vi "find next node.vi"(8 "error in (no error)":errorcluster, 10 "map":T1[][](array[typedef]), 11 "current_path in":T1[](array[typedef])) -> (0 "error out":errorcluster, 1 "T = a next node was found":bool, 2 "next node":T1, 3 "current_path out":T1[](array[typedef]))   [LabVIEW 2021, in "Project Euler.lvlib"]
uses:
  Project Euler.lvlib
  lattice_path_node.ctl
  lattice_path_direction.ctl
panel:
  out "map no. of columns":i32
  out "map no. of rows":i32
  out "last (most recent) node of path":T1
  # "Development\ncontrols/indicators useful for development and testing, but which are not outputs of the VI"
  # "Input\nInputs to the VI"
  # "Output\nOutputs of the VI"
  # "Description\n\nBlank VI with error handling case. \n\nSummarize the use of this VI in this space."
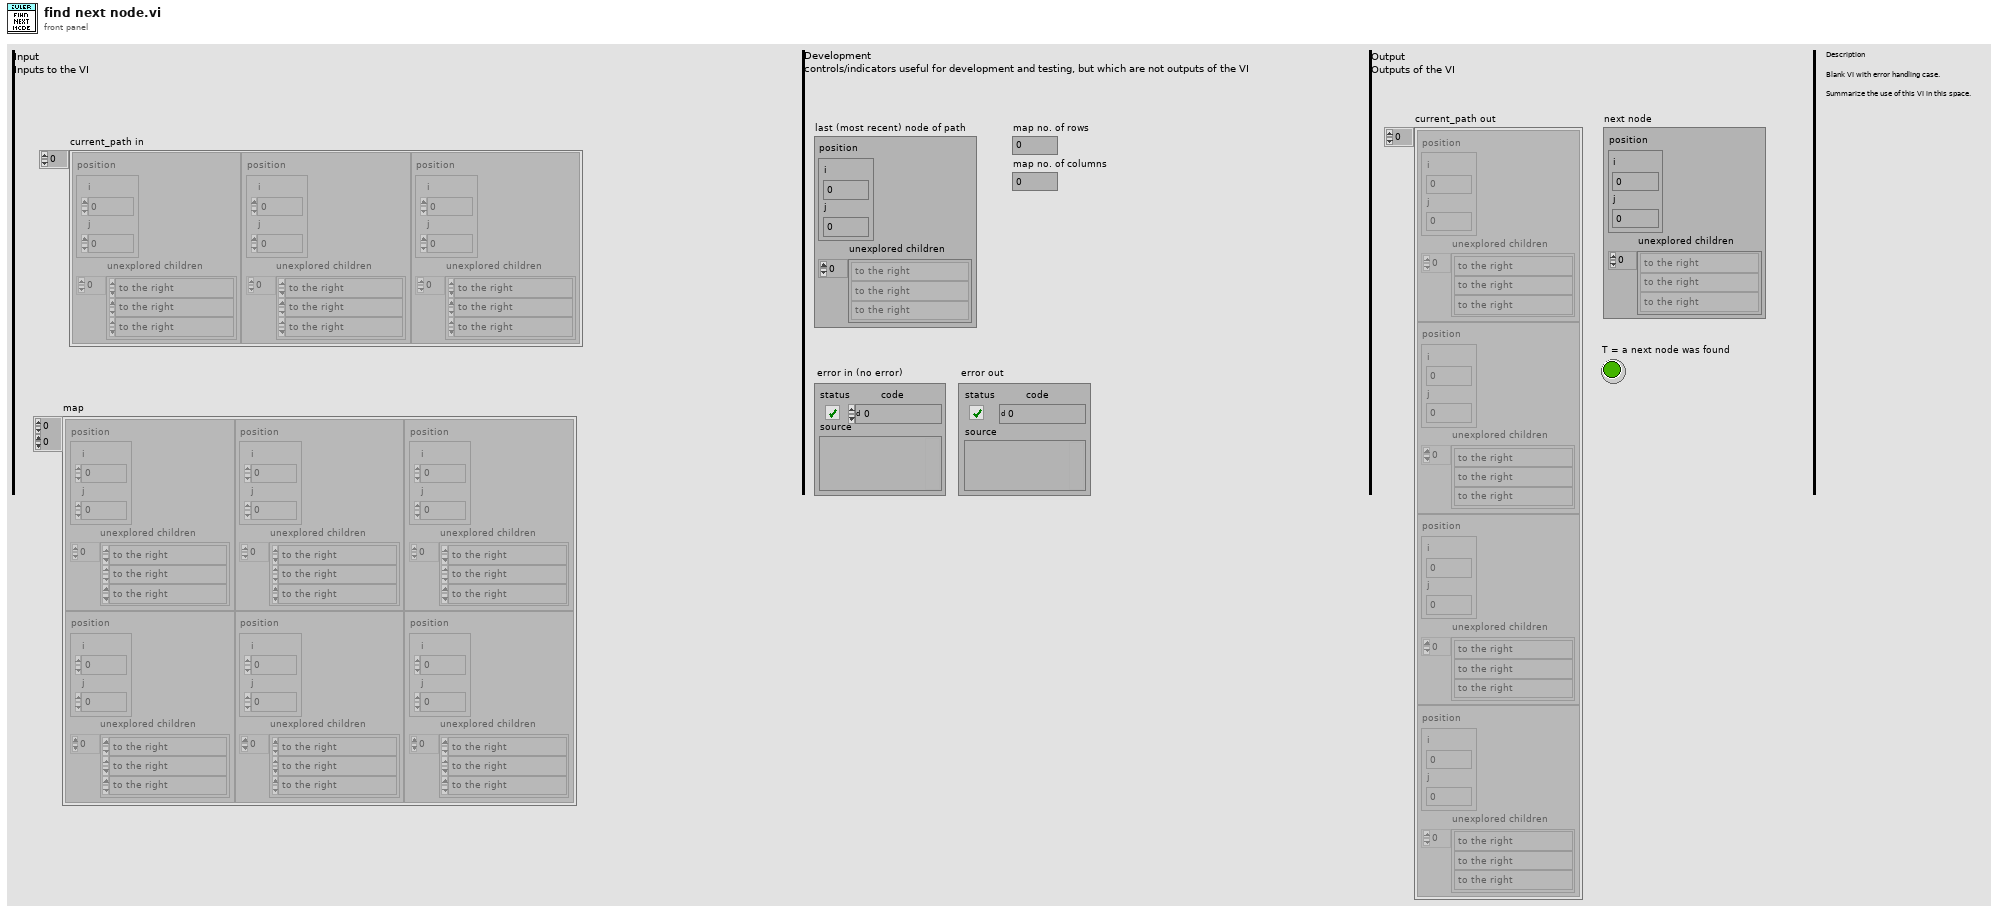
[diagram p1: front panel]
types:
  T1 = typedef "Project Euler.lvlib/lattice_path_node.ctl" = cluster{"position":cluster{"i":i32, "j":i32}, "unexplored children":T2[]}
  T2 = typedef "Project Euler.lvlib/lattice_path_direction.ctl" = enum16{"to the right", "downwards"}
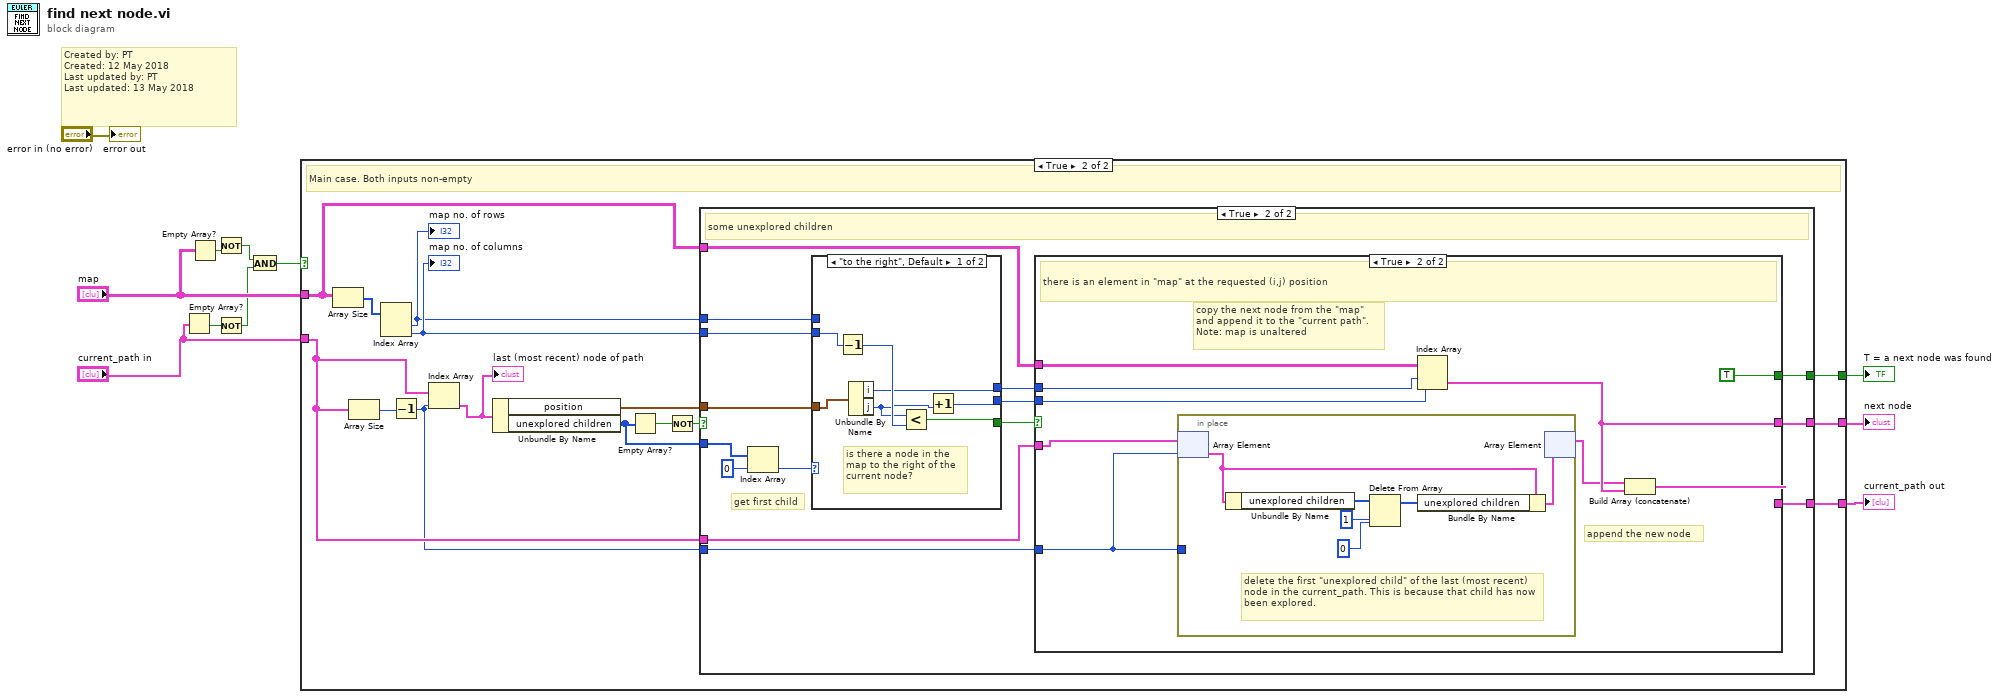
[diagram p0: block diagram]
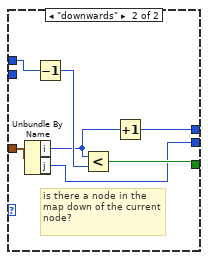
[diagram p5: hidden frame]
diagram:
  # "Created by: PT\nCreated: 12 May 2018\nLast updated by: PT\nLast updated: 13 May 2018"
  n1 = Empty Array?(array="current_path in") -> (empty?=w7:bool)
  n2 = Empty Array?(array="map") -> (empty?=w10:bool)
  n3 = Not(x=w10) -> (.not. x?=w5:bool)
  n4 = Not(x=w7) -> (.not. x?=w6:bool)
  n5 = And(x=w5, y=w6) -> (x .and. y?=w4:bool)
  n6 = case shown="True" w4 {
    tunnel: "map" -> [_ w18]
    tunnel: "current_path in" -> [w12 w16]
    tunnel: [_ w17] -> w3
    tunnel: [w12 w14] -> w2
    tunnel: [_ w13] -> w1
    frame False {
      # "Corner case. map OR current_path are empty."
    }
    frame True {
      # "Main case. Both inputs non-empty"
      n7 = Array Size(array=w18) -> (size(s)=w21:i32[])
      n8 = Array Size(array=w16) -> (size(s)=w27:i32)
      n9 = Index Array(array=w21) -> (element #1=w19:i32, element #2=w20:i32)  [unwired: 2 in]
      "map no. of rows" <- w19
      "map no. of columns" <- w20
      n10 = Decrement(x=w27) -> (x-1=w15:i32)
      n11 = Index Array(array=w16, index=w15) -> (element=w26:T1)
      "last (most recent) node of path" <- w26
      n12 = Unbundle By Name(w26) -> ("position"=w23:cluster{"i":i32, "j":i32}, "unexplored children"=w22:T2[])
      n13 = Empty Array?(array=w22) -> (empty?=w25:bool)
      n14 = Not(x=w25) -> (.not. x?=w24:bool)
      n15 = case shown="True" w24 {
        tunnel: w23 -> [_ w40]
        tunnel: w22 -> [_ w43]
        tunnel: w20 -> [_ w39]
        tunnel: w19 -> [_ w38]
        tunnel: w18 -> [_ w34]
        tunnel: [_ w33] -> w17
        tunnel: w16 -> [w28 w32]
        tunnel: w15 -> [_ w31]
        tunnel: [w28 w30] -> w14
        tunnel: [_ w29] -> w13
        frame False {
          # "all children are explored already"
        }
        frame True {
          # "get first child"
          # "some unexplored children"
          n16 = Index Array(array=w43, index=0) -> (element=w41:T2)
          n17 = case shown="\"to the right\", Default" w41 {
            tunnel: w40 -> [w66 w73]
            tunnel: w39 -> [w65 _]
            tunnel: w38 -> [_ w72]
            tunnel: [w63 w70] -> w37
            tunnel: [w62 w68] -> w36
            tunnel: [w60 w67] -> w35
            frame "to the right", Default {
              # "is there a node in the map to the right of the current node?"
              n18 = Decrement(x=w65) -> (x-1=w64:i32)
              n19 = Unbundle By Name(w66) -> ("i"=w62:i32, "j"=w61:i32)
              n20 = Less?(x=w61, y=w64) -> (x < y?=w63:bool)
              n21 = Increment(x=w61) -> (x+1=w60:i32)
            }
            frame "downwards" {
              # "is there a node in the map down of the current node?"
              n22 = Unbundle By Name(w73) -> ("i"=w69:i32, "j"=w67:i32)
              n23 = Decrement(x=w72) -> (x-1=w71:i32)
              n24 = Less?(x=w69, y=w71) -> (x < y?=w70:bool)
              n25 = Increment(x=w69) -> (x+1=w68:i32)
            }
          }
          n26 = case shown="True" w37 {
            tunnel: w36 -> [_ w52]
            tunnel: w35 -> [_ w51]
            tunnel: w34 -> [_ w53]
            tunnel: [_ w50] -> w33
            tunnel: w32 -> [w44 w45]
            tunnel: w31 -> [_ w47]
            tunnel: [w44 w49] -> w30
            tunnel: [_ TRUE] -> w29
            frame False {
              # "child of last (most recent) node is outside map"
            }
            frame True {
              # "copy the next node from the \"map\" and append it to the \"current path\". Note: map is unaltered"
              # "append the new node"
              # "there is an element in \"map\" at the requested (i,j) position"
              n27 = in-place {
                in-place-border: w47 -> [_]
                # "delete the first \"unexplored child\" of the last (most recent) node in the current_path. This is because that child has now been explored."
                n28 = in-place-array #1(w45, w47) -> (w54:T1)
                n29 = Unbundle By Name(w54) -> ("unexplored children"=w59:T2[])
                n30 = Delete From Array(array=w59, length=1, index=0) -> (array with subset deleted=w58:T2[])  [unwired: 1 out]
                n31 = Bundle By Name(cluster=w54, "unexplored children"=w58) -> (w55:T1)
                n32 = in-place-array #1(w55) -> (w46:T1[])  [unwired: 1 out]
              }
              n33 = Index Array(array=w53, index (row)=w52, index (col)=w51) -> (element=w50:T1)
              n34 = Build Array (concatenate)(w46, w50) -> (w49:T1[])
            }
          }
        }
      }
    }
  }
  "T = a next node was found" <- w1
  "current_path out" <- w2
  "next node" <- w3
  "error out" <- "error in (no error)"
